vi "setText.vi"(0 "reference":refnum<class "MultiLineString.lvclass">, 1 "text":string, 5 "error in (no error)":errorcluster) -> (14 "reference out":refnum<class "MultiLineString.lvclass">, 19 "error out":errorcluster)   [LabVIEW 2014, in "MultiLineString.lvclass"]
doc: "public void setText(String newValue)"
uses:
  <resource>/Framework/Providers/Open_GDS/UML/MultiLineString_class/MultiLineString.lvclass
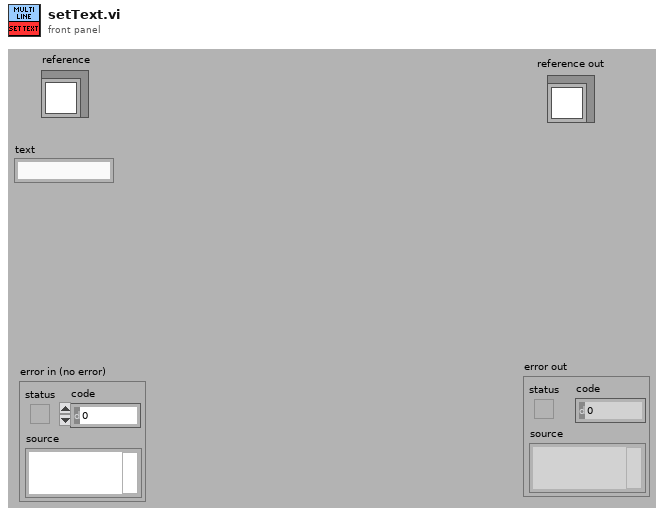
[diagram p1: front panel]
types:
  T1 = typedef "MultiLineString.lvclass/ObjectAttributes.ctl" = cluster{"GAP":i32, "text":string, "justification":T2, "size":T3, "underlined":bool}
  T2 = typedef "MultiLineString.lvclass/JustificationType.ctl" = enum16{"LEFT", "CENTER", "RIGHT"}
  T3 = typedef "MultiLineString.lvclass/SizeType.ctl" = enum16{"LARGE", "NORMAL", "SMALL"}
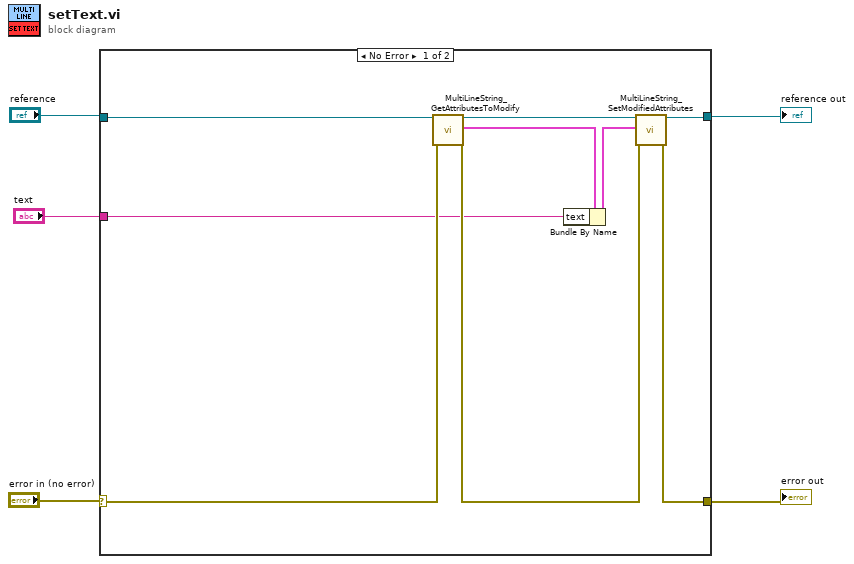
[diagram p0: block diagram]
diagram:
  n1 = case shown="No Error" "error in (no error)" {
    selector: "error in (no error)" -> [w14 w15]
    tunnel: "reference" -> [w13 w16]
    tunnel: [w8 w15] -> w2
    tunnel: [w7 w16] -> w3
    tunnel: "text" -> [w6 _]
    frame No Error {
      n2 = call <resource>:"MultiLineString_GetAttributesToModify.vi"("reference in"=w13, "error in (no error)"=w14) -> ("reference out"=w11:refnum<class "MultiLineString.lvclass">, "Attributes"=w10:T1, "error out"=w12:errorcluster)  [unwired: 1 in, 14 out]
      n3 = Bundle By Name(cluster=w10, "text"=w6) -> (w9:T1)
      n4 = call <resource>:"MultiLineString_SetModifiedAttributes.vi"("reference in"=w11, "Attributes"=w9, "error in (no error)"=w12) -> ("reference out"=w7:refnum<class "MultiLineString.lvclass">, "error out"=w8:errorcluster)  [unwired: 3 in, 12 out]
    }
    frame Error {
    }
  }
  "reference out" <- w3
  "error out" <- w2
